vi "Bode_diag.vi"() -> ()   [LabVIEW 2015]
panel:
  out "Frequency":dbl
  in  "End Freq":dbl
  in  "Start freq":dbl
  in  "Freq pts":i32=100
  out "XY Graph 2":cluster{dbl[], dbl[]}(graph)
  out "XY Graph":cluster{dbl[], dbl[]}(graph)
  out "phase":dbl
  out "amplitude":dbl
  in  "error in":errorcluster
  in  "address string":string="4"
  in  "stop":bool
  in  "Measure":bool
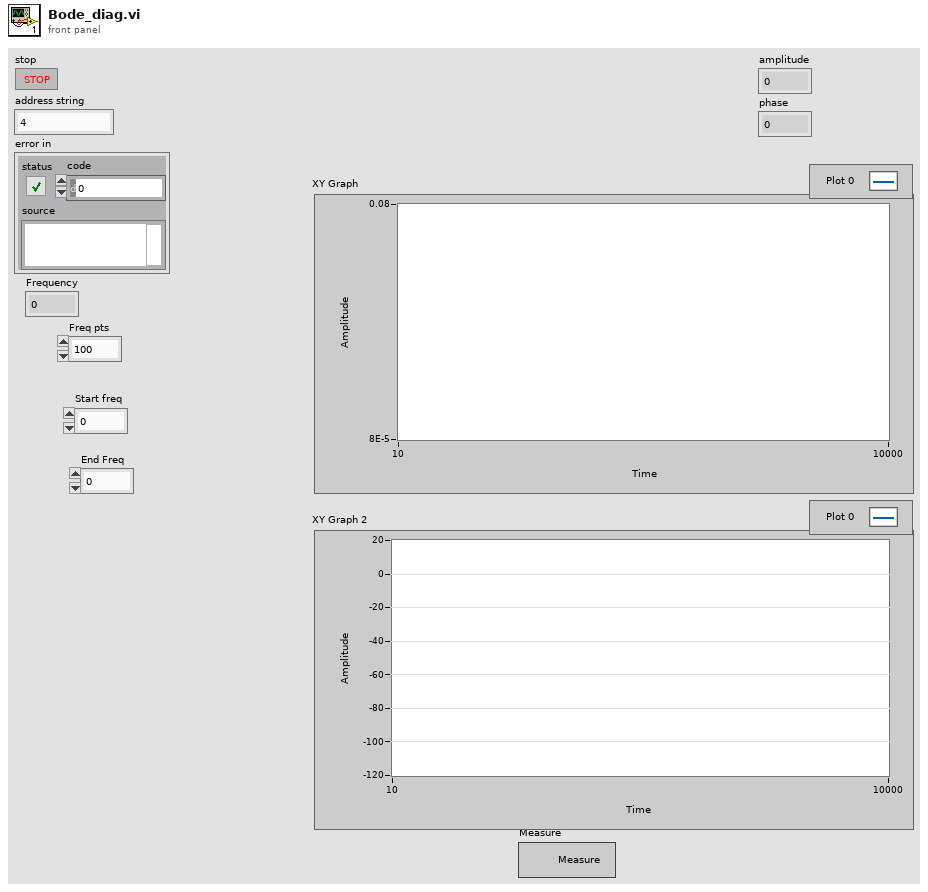
[diagram p1: front panel]
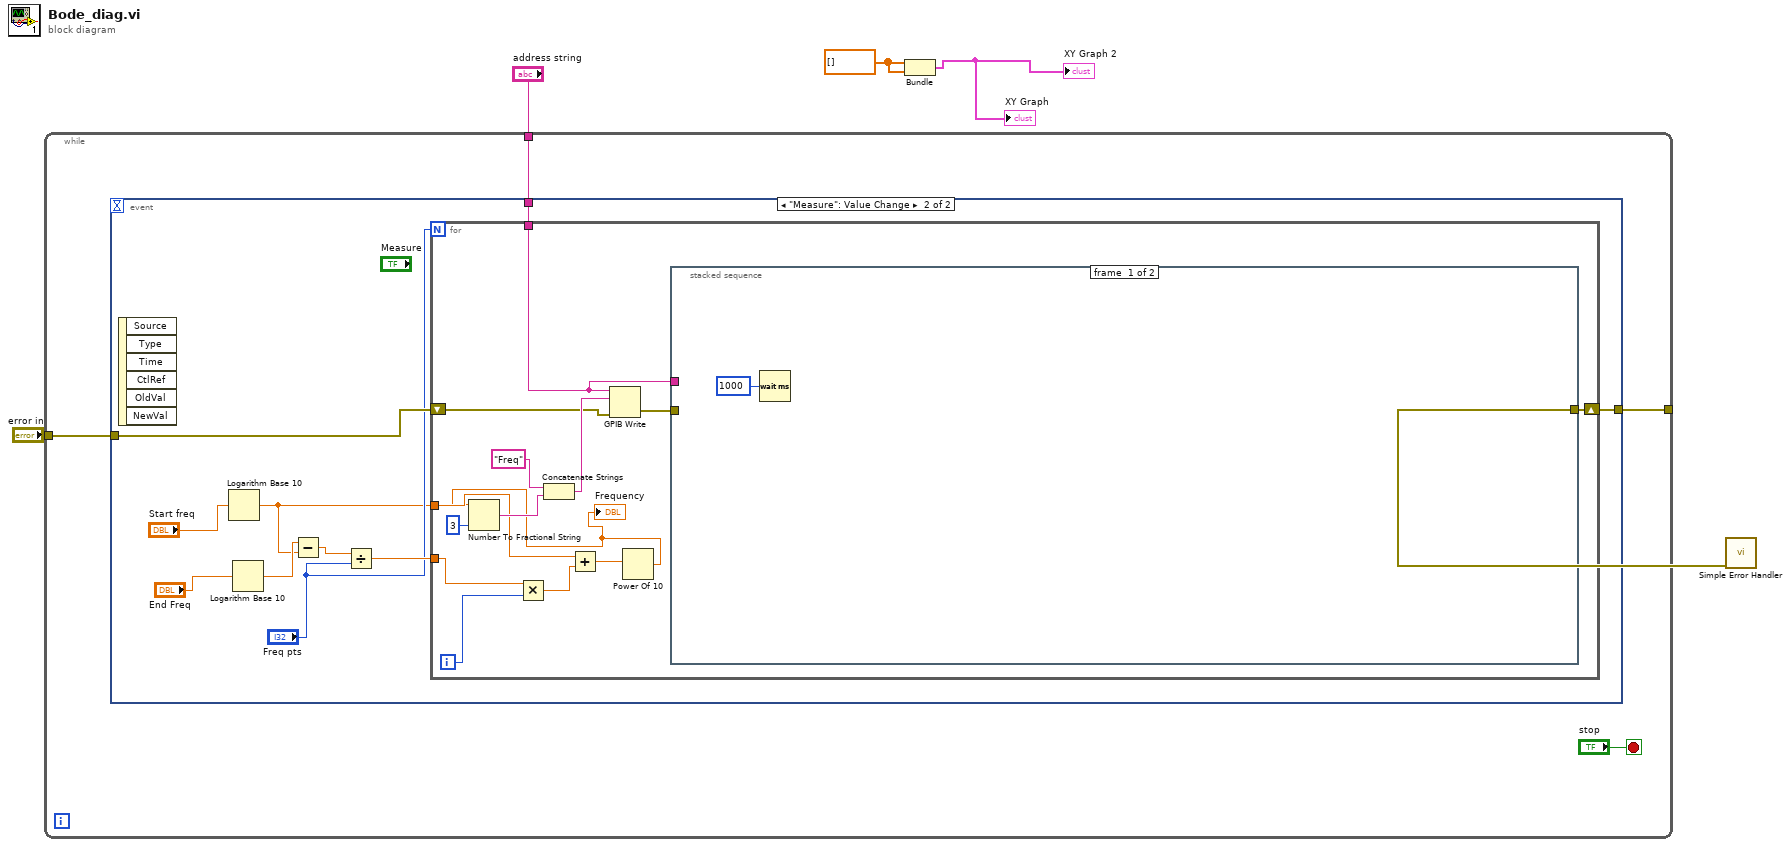
[diagram p0: block diagram]
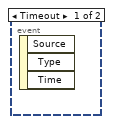
[diagram p2: hidden frame]
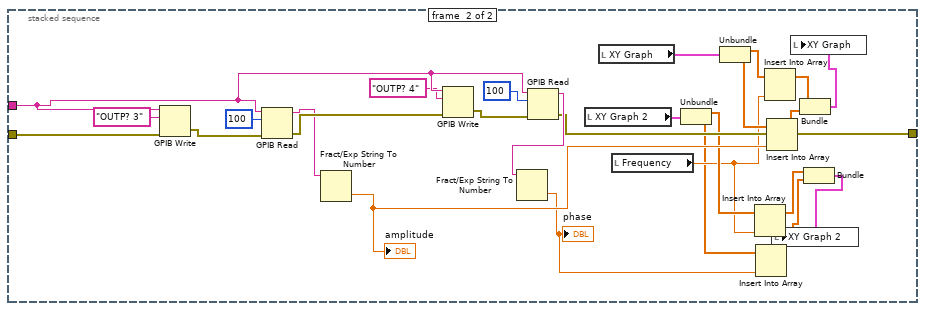
[diagram p3: hidden frame]
diagram:
  w2 = dbl[] []
  n1 = while {
    tunnel: "error in" -> [w8]
    tunnel: [w7] -> w4
    tunnel: "address string" -> [w6]
    stop <- "stop" stop-if-true
    n2 = event shown="[1] \"Measure\": Value Change" {
      selector: _ -> [_ _]
      dyn-events: _ -> [_ _]
      timeout: _ -> [_ _]
      tunnel: w8 -> [_ w19]
      tunnel: [_ w18] -> w7
      tunnel: w6 -> [_ w17]
      event Timeout {
        n3 = event-data() -> ()  [unwired: 1 in, 3 out]
      }
      event "Measure": Value Change {
        n4 = event-data() -> ()  [unwired: 1 in, 6 out]
        n5 = Logarithm Base 10(1:"Start freq") -> (0:w10:dbl)
        n6 = Logarithm Base 10(1:"End Freq") -> (0:w11:dbl)
        n7 = Subtract(x=w11, y=w10) -> (x-y=w16:dbl)
        n8 = Divide(x=w16, y="Freq pts") -> (x/y=w13:dbl)
        n9 = for {
          N: "Freq pts" -> [_]
          tunnel: w17 -> [w26]
          shift-right: [w27] -> w18
          shift-left: w19 -> [w28]
          tunnel: w13 -> [w23]
          tunnel: w10 -> [w24]
          i -> [w22]
          n10 = Multiply(x=w23, y=w22) -> (x*y=w25:dbl)
          n11 = Add(x=w24, y=w25) -> (x+y=w21:dbl)
          n12 = Power Of 10(x=w21) -> (10^x=w20:dbl)
          "Frequency" <- w20
          n13 = Number To Fractional String(number=w20, precision (6)=i16 3) -> (F-format string=w31:string)  [unwired: 2 in]
          n14 = Concatenate Strings("Freq" ("string"), w31) -> (w30:string)
          n15 = GPIB Write(0:w26, 1:w30, 3:w28) -> (6:w29:errorcluster)  [unwired: 2 in, 1 out]
          n16 = stacked-sequence {
            tunnel: w29 -> [_ w60]
            tunnel: w26 -> [_ w51]
            tunnel: [_ w52] -> w27
            frame #0 {
              n17 = Wait (ms)(milliseconds to wait=u32 1000) -> ()  [unwired: 1 out]
            }
            frame #1 {
              n18 = GPIB Write(0:w51, 1:"OUTP? 3" ("data"), 3:w60) -> (6:w59:errorcluster)  [unwired: 2 in, 1 out]
              n19 = GPIB Read(0:w51, 1:100 ("byte count"), 3:w59) -> (5:w54:string, 7:w57:errorcluster)  [unwired: 2 in, 1 out]
              n20 = Fract/Exp String To Number(string=w54) -> (number=w45:dbl)  [unwired: 3 in, 1 out]
              "amplitude" <- w45
              n21 = GPIB Write(0:w51, 1:"OUTP? 4" ("data"), 3:w57) -> (6:w56:errorcluster)  [unwired: 2 in, 1 out]
              n22 = GPIB Read(0:w51, 1:100 ("byte count"), 3:w56) -> (5:w53:string, 7:w52:errorcluster)  [unwired: 2 in, 1 out]
              n23 = Fract/Exp String To Number(string=w53) -> (number=w41:dbl)  [unwired: 3 in, 1 out]
              "phase" <- w41
              n24 = local read "XY Graph 2"() -> (w48:cluster{dbl[], dbl[]})
              n25 = local read "XY Graph"() -> (w49:cluster{dbl[], dbl[]})
              n26 = local read "Frequency"() -> (w43:dbl)
              n27 = Unbundle(w48) -> (w44:dbl[], w42:dbl[])
              n28 = Unbundle(w49) -> (w47:dbl[], w46:dbl[])
              n29 = Insert Into Array(array=w44, new element=w43) -> (w37:dbl[])  [unwired: 1 in]
              n30 = Insert Into Array(array=w42, new element=w41) -> (w36:dbl[])  [unwired: 1 in]
              n31 = Insert Into Array(array=w47, new element=w43) -> (w40:dbl[])  [unwired: 1 in]
              n32 = Insert Into Array(array=w46, new element=w45) -> (w39:dbl[])  [unwired: 1 in]
              n33 = Bundle(w40, w39) -> (w38:cluster{dbl[], dbl[]})  [unwired: 1 in]
              n34 = local write "XY Graph"(w38) -> ()
              n35 = Bundle(w37, w36) -> (w35:cluster{dbl[], dbl[]})  [unwired: 1 in]
              n36 = local write "XY Graph 2"(w35) -> ()
            }
          }
        }
      }
    }
  }
  n37 = Bundle(w2, w2) -> (→"XY Graph" →"XY Graph 2":cluster{dbl[], dbl[]})  [unwired: 1 in]
  n38 = call <vilib>:"Simple Error Handler.vi"("error in (no error)"=w4) -> ()  [unwired: 4 in, 5 out]
